vi "mks946_get_pressure_unit.vi"(6 "err_in":errorcluster, 7 "visa_in":refnum<visa-resource-name>="COM3", 11 "address":i32=253) -> (0 "status":bool=TRUE, 2 "message":string, 4 "err_out":errorcluster, 5 "visa_out":refnum<visa-resource-name>="COM3")   [LabVIEW 2019]
panel:
  out "full_scale":string
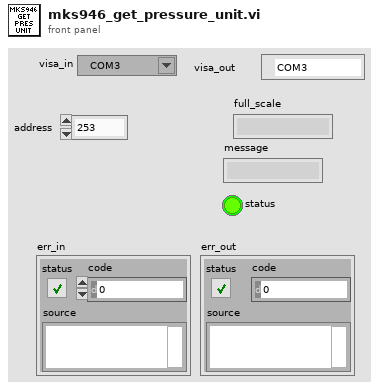
[diagram p1: front panel]
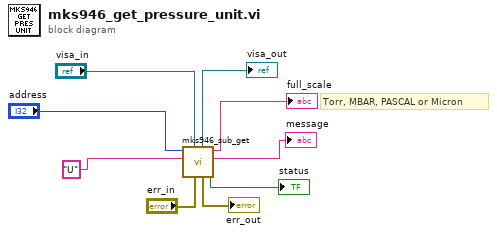
[diagram p0: block diagram]
diagram:
  # "Torr, MBAR, PASCAL or Micron"
  n1 = call "mks946_sub_get.vi"("error in (no error)"="err_in", "VISA_ref_in"="visa_in", "command"="U" ("mks946_comm"), "address"="address") -> ("status"=→"status":bool, "message"=→"message":string, "response"=→"full_scale":string, "error out"=→"err_out":errorcluster, "VISA_ref_out"=→"visa_out":refnum<visa-resource-name>)  [unwired: 3 in]
